vi "CaptureWindowImage.vi"(8 "Error in":errorcluster, 9 "File Path":path, 11 "Window Name":string) -> (0 "error out":errorcluster)   [LabVIEW 2013]
doc: "Chwcking the existence of given named Vi in memory and coonverting it to VI Refernce if existing or else throwing an error 123"
uses:
  C:/Windows/System32/user32.dll
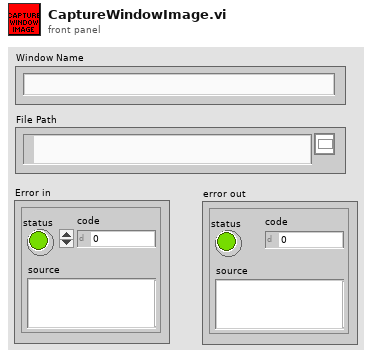
[diagram p1: front panel]
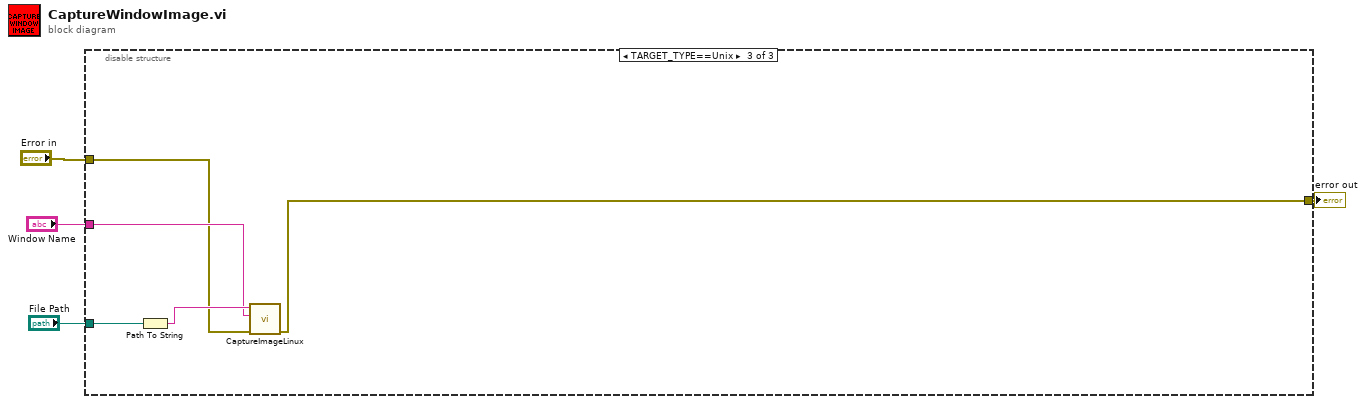
[diagram p0: block diagram]
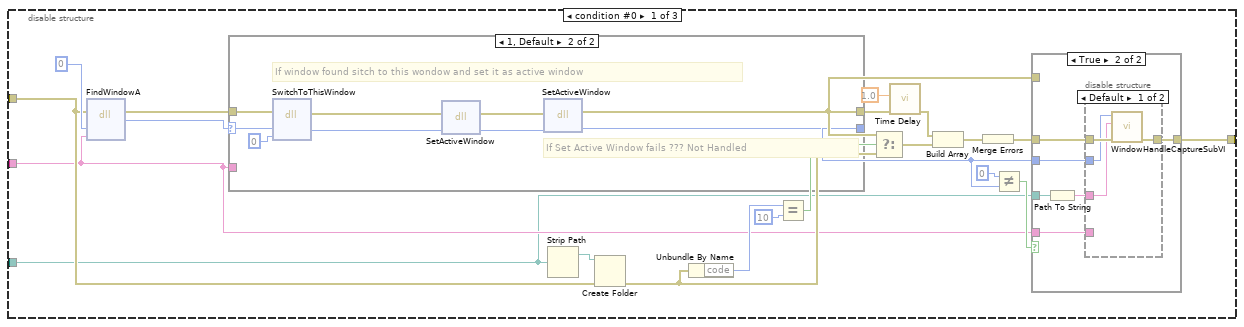
[diagram p2: hidden frame]
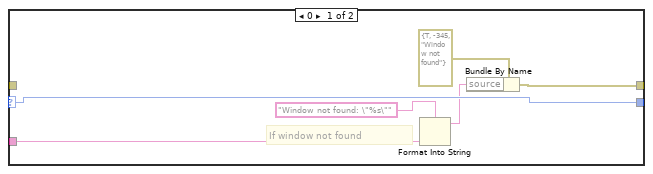
[diagram p3: hidden frame]
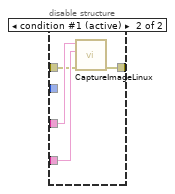
[diagram p5: hidden frame]
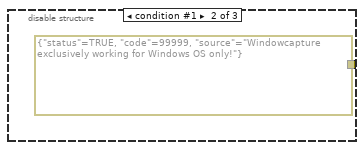
[diagram p6: hidden frame]
diagram:
  n1 = disable-structure shown="TARGET_TYPE==Unix" {
    disable-tunnel: [w13 errorcluster {"status"=TRUE, "code"=99999, "source"="Windowcapture exclusively working for Windows OS only!"} ("error out") w57] -> w4
    disable-tunnel: "Error in" -> [w9 _ w58]
    disable-tunnel: "Window Name" -> [w6 _ w59]
    disable-tunnel: "File Path" -> [w5 _ w61]
    frame condition #0 {
      n2 = dll-call lib="C:/Windows/System32/user32.dll" fn="FindWindowA"(error in=w9, "Class Name"=0, "Window Name"=w6) -> (error out=w11:errorcluster, "Handle"=w12:i32)  [unwired: 4 in, 1 out]
      n3 = case shown="1, Default" w12 {
        selector: w12 -> [w31 w36]
        tunnel: [w31 w39] -> w7
        tunnel: w11 -> [_ w38]
        tunnel: [w27 w37] -> w8
        tunnel: w6 -> [w26 _]
        frame 0 {
          # "If window not found"
          n4 = Format Into String(format string="Window not found: \"%s\"" ("source"), w26) -> (resulting string=w30:string)  [unwired: 2 in, 1 out]
          n5 = Bundle By Name(cluster=errorcluster {"status"=TRUE, "code"=-345, "source"="Window not found"} ("error out"), "source"=w30) -> (w27:errorcluster)
        }
        frame 1, Default {
          # "If Set Active Window fails ??? Not Handled"
          # "If window found sitch to this wondow and set it as active window"
          n6 = dll-call lib="C:/Windows/System32/user32.dll" fn="SwitchToThisWindow"(error in=w38, "Handle"=w36, "Boolean"=i8 0) -> (error out=w34:errorcluster, "Handle"=w33:i32)  [unwired: 3 in, 2 out]
          n7 = dll-call lib="C:/Windows/System32/user32.dll" fn="SetActiveWindow"(error in=w34, "Handle"=w33) -> (error out=w35:errorcluster, "Handle"=w32:i32)  [unwired: 2 in, 2 out]
          n8 = dll-call lib="C:/Windows/System32/user32.dll" fn="SetActiveWindow"(error in=w35, "Handle"=w32) -> (error out=w37:errorcluster, "Handle"=w39:i32)  [unwired: 2 in, 2 out]
        }
      }
      n9 = Strip Path(path=w5) -> (stripped path=w22:path)  [unwired: 1 out]
      n10 = Create Folder(path (use dialog)=w22, error in=w9) -> (error out=w14:errorcluster)  [unwired: 3 out]
      n11 = Unbundle By Name(w14) -> ("code"=w21:i32)
      n12 = Equal?(x=w21, y=10) -> (x = y?=w19:bool)
      n13 = Select(t=w8, s=w19, f=w14) -> (s? t:f=w17:errorcluster)
      n14 = call "Time Delay"("error in (no error)"=w8, "Delay Time (s)"=1.0) -> ("error out"=w18:errorcluster)  [unwired: 9 out]
      n15 = Build Array(w18, w17) -> (w15:errorcluster[])
      n16 = Merge Errors(w15) -> (w16:errorcluster)
      n17 = Not Equal?(x=0 ("y"), y=w7) -> (x != y?=w24:bool)
      n18 = case shown="True" w24 {
        tunnel: w8 -> [_ _]
        tunnel: [w41 w45] -> w13
        tunnel: w7 -> [_ w46]
        tunnel: w16 -> [w41 w44]
        tunnel: w6 -> [_ w43]
        tunnel: w5 -> [_ w42]
        frame False {
        }
        frame True {
          n19 = Path To String(path=w42) -> (string=w47:string)
          n20 = disable-structure shown="Default" {
            disable-tunnel: w47 -> [w49 w55]
            disable-tunnel: w46 -> [w48 _]
            disable-tunnel: [w50 w52] -> w45
            disable-tunnel: w44 -> [w51 w53]
            disable-tunnel: w43 -> [_ w54]
            frame condition #0 {
              n21 = call "WindowHandleCaptureSubVI.vi"("error in (no error)"=w51, "Path"=w49, "Handle"=w48) -> ("error out"=w50:errorcluster)  [unwired: 8 in]
            }
            frame condition #1 (active) {
              n22 = call "CaptureImageLinux.vi"("error in"=w53, "WindowName"=w54, "PathWheretoSave"=w55) -> ("error out"=w52:errorcluster)  [unwired: 8 in]
            }
          }
        }
      }
    }
    frame condition #1 {
    }
    frame condition #2 (active) {
      n23 = Path To String(path=w61) -> (string=w60:string)
      n24 = call "CaptureImageLinux.vi"("error in"=w58, "WindowName"=w59, "PathWheretoSave"=w60) -> ("error out"=w57:errorcluster)  [unwired: 8 in]
    }
  }
  "error out" <- w4
